vi "Convert To 2D Array.vi"(8 "error in (no error)":errorcluster, 9 "Name":string, 10 "TableName":string, 11 "ExcuseNotesHandler":refnum<class "ExcuseNotesHandler.lvclass">) -> (0 "error out":errorcluster, 2 "2D Array":string[][](array[string]), 3 "ExcuseNotesHandler Out":refnum<class "ExcuseNotesHandler.lvclass">)   [LabVIEW 2015, in "ExcuseNotesHandler.lvclass"]
uses:
  ExcuseNotesHandler.lvclass
  Global Variable/g_Pos_Determine.vi
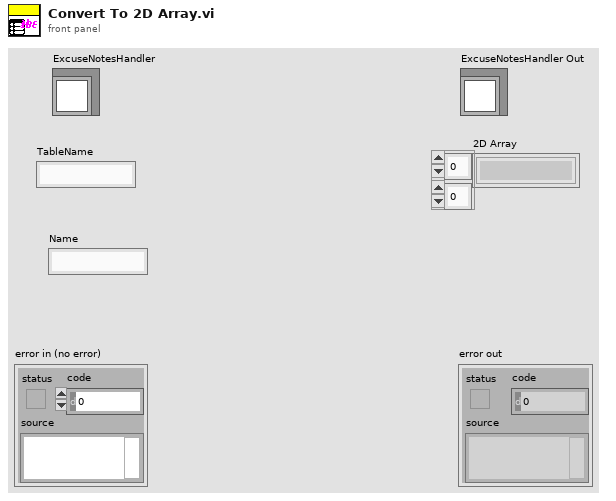
[diagram p1: front panel]
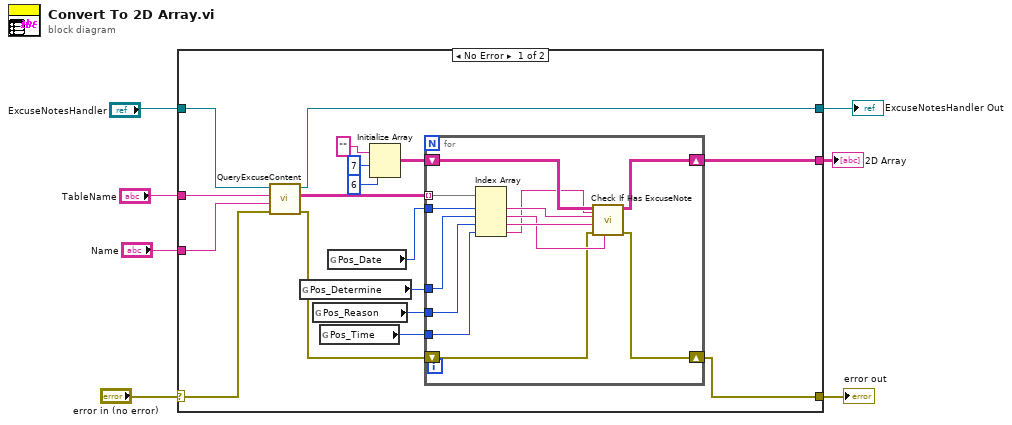
[diagram p0: block diagram]
diagram:
  n1 = case shown="No Error" "error in (no error)" {
    selector: "error in (no error)" -> [w21 w39]
    tunnel: [w9 w39] -> w6
    tunnel: [w20 w38] -> w4
    tunnel: "ExcuseNotesHandler" -> [w24 w38]
    tunnel: "TableName" -> [w23 _]
    tunnel: "Name" -> [w22 _]
    tunnel: [w8 _] -> w1
    frame No Error {
      n2 = call "QueryExcuseContent.vi"("error in (no error)"=w21, "Name"=w22, "TableName"=w23, "ExcuseNotesHandler"=w24) -> ("error out"=w10:errorcluster, "ExcuseNote(\"\")"=w19:string[][], "ExcuseNotesHandler Out"=w20:refnum<class "ExcuseNotesHandler.lvclass">)  [unwired: 5 in]
      n3 = global read "g_Pos_Determine.vi" "Pos_Determine"() -> (w13:i32)
      n4 = global read "g_Pos_Determine.vi" "Pos_Reason"() -> (w12:i32)
      n5 = global read "g_Pos_Determine.vi" "Pos_Time"() -> (w11:i32)
      n6 = global read "g_Pos_Determine.vi" "Pos_Date"() -> (w14:i32)
      n7 = Initialize Array("", 7 ("dimension size"), 6 ("dimension size")) -> (w15:string[][])
      n8 = for {
        tunnel: w19 -> [w37] mode=indexing
        shift-right: [w25] -> w8
        shift-left: w15 -> [w34]
        tunnel: w14 -> [w36]
        tunnel: w13 -> [w35]
        tunnel: w12 -> [w33]
        tunnel: w11 -> [w29]
        shift-right: [w26] -> w9
        shift-left: w10 -> [w27]
        n9 = Index Array(array=w37, index #1=w36, index #2=w35, index #3=w33, index #4=w29) -> (element #1=w30:string, element #2=w31:string, element #3=w32:string, element #4=w28:string)
        n10 = call "Check If Has ExcuseNote.vi"("Determine(\"\")"=w31, "Time(\"\")"=w28, "error in (no error)"=w27, "ExcuseNote(\"\")"=w32, "Date"=w30, "List"=w34) -> ("error out"=w26:errorcluster, "2D Array"=w25:string[][])  [unwired: 4 in]
      }
    }
    frame Error {
    }
  }
  "error out" <- w6
  "ExcuseNotesHandler Out" <- w4
  "2D Array" <- w1
